vi "Format ECU Master Key to String.vi"(11 "Data":dbl[](array[numeric])) -> (3 "string":string)   [LabVIEW 2024, in "Diagnostics Addon Shared.lvlib"]
uses:
  Diagnostics Addon Shared.lvlib
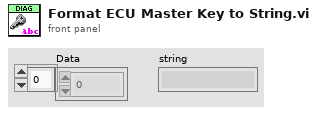
[diagram p1: front panel]
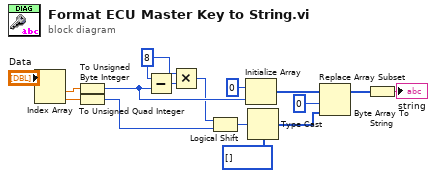
[diagram p0: block diagram]
diagram:
  w16 = 8 ("x")
  n1 = Index Array(array="Data") -> (element #1=w3:dbl, element #2=w1:dbl)  [unwired: 2 in]
  n2 = To Unsigned Byte Integer(number=w3) -> (unsigned 8bit integer=w13:u8)
  n3 = To Unsigned Quad Integer(1:w1) -> (0:w14:u64)
  n4 = Subtract(x=w16, y=w13) -> (x-y=w11:i32)
  n5 = Multiply(x=w16, y=w11) -> (x*y=w12:i32)
  n6 = Logical Shift(y=w12, x=w14) -> (x << y=w10:u64)
  n7 = Initialize Array(u8 0, w13) -> (w6:u8[])
  n8 = Type Cast(type=u8[] [], x=w10) -> (*(type *) &x=w7:u8[])
  n9 = Replace Array Subset(array=w6, new element=w7, index=0) -> (w9:u8[])
  n10 = Byte Array To String(unsigned byte array=w9) -> (string=→"string":string)
